vi "BlynkLogs.vi"() -> ()   [LabVIEW 2014]
panel:
  in  "BlynkLogs":string[](array[string])
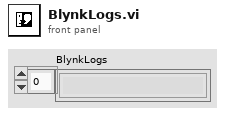
[diagram p1: front panel]
diagram:
